vi "VITester - VI Tree.vi"() -> ()   [LabVIEW 2013]
panel:
  in  "Boolean":bool
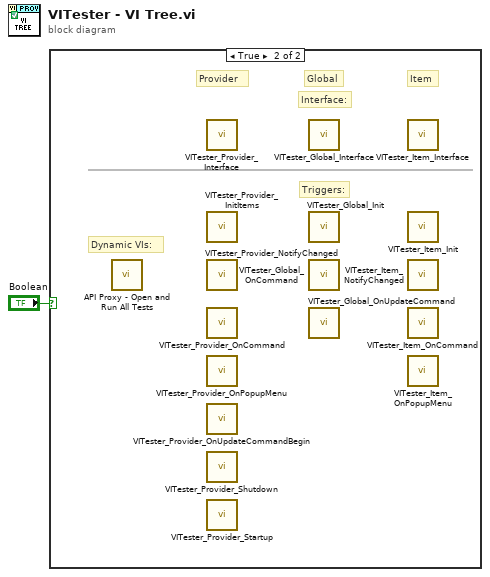
[diagram p0: block diagram]
diagram:
  n1 = case shown="True" "Boolean" {
    frame False {
    }
    frame True {
      # "Dynamic VIs:"
      # "Triggers:"
      # "Interface:"
      # "Item"
      # "Global"
      # "Provider"
      n2 = call <resource>:"API Proxy - Open and Run All Tests.vi"() -> ()  [unwired: 1 in]
      n3 = call <resource>:"VITester_Provider_Interface.vi"() -> ()  [unwired: 11 in, 1 out]
      n4 = call <resource>:"VITester_Provider_InitItems.vi"() -> ()  [unwired: 12 in]
      n5 = call <resource>:"VITester_Provider_NotifyChanged.vi"() -> ()  [unwired: 11 in, 1 out]
      n6 = call <resource>:"VITester_Provider_OnCommand.vi"() -> ()  [unwired: 12 in]
      n7 = call <resource>:"VITester_Provider_OnPopupMenu.vi"() -> ()  [unwired: 12 in]
      n8 = call <resource>:"VITester_Provider_OnUpdateCommandBegin.vi"() -> ()  [unwired: 12 in]
      n9 = call <resource>:"VITester_Provider_Shutdown.vi"() -> ()  [unwired: 11 in, 1 out]
      n10 = call <resource>:"VITester_Provider_Startup.vi"() -> ()  [unwired: 11 in, 1 out]
      n11 = call <resource>:"VITester_Global_Interface.vi"() -> ()  [unwired: 11 in, 1 out]
      n12 = call <resource>:"VITester_Global_Init.vi"() -> ()  [unwired: 12 in]
      n13 = call <resource>:"VITester_Global_OnCommand.vi"() -> ()  [unwired: 12 in]
      n14 = call <resource>:"VITester_Global_OnUpdateCommand.vi"() -> ()  [unwired: 11 in, 1 out]
      n15 = call <resource>:"VITester_Item_Interface.vi"() -> ()  [unwired: 11 in, 1 out]
      n16 = call <resource>:"VITester_Item_Init.vi"() -> ()  [unwired: 12 in]
      n17 = call <resource>:"VITester_Item_NotifyChanged.vi"() -> ()  [unwired: 11 in, 1 out]
      n18 = call <resource>:"VITester_Item_OnCommand.vi"() -> ()  [unwired: 12 in]
      n19 = call <resource>:"VITester_Item_OnPopupMenu.vi"() -> ()  [unwired: 12 in]
    }
  }
